vi "Tree Map to Tree Control Items.vi"(7 "Preserve Insertion Order? (F)":bool, 11 "Tree Map In":T2) -> (3 "Tree Control Items":T1(array[cluster]))   [LabVIEW 2020, in "Tree Map.lvlib"]
doc: "Translates the Tree Map representation into Tree Control Elements.\n\n<b>NOTE</b> - The order of elements is defined in alphabetical order, due to the implementation of Sets and Maps in LabVIEW. This effect only appears if there are 1M+ nodes with the same name under the same parent node. \nIf a different order of visualization is required, the user needs to access the array of Tree Control elements returned by this function and reorder the items using a custom algorithm.\n\n<b>Author:</b> Piotr Kruczkowski <PrimaryKey>\n<b>License:</b> NewBSD\n\nCopyright (c) 2019, National Instruments\nAll rights reserved.\n\nRedistribution and use in source and binary forms, with or without\nmodification, are permitted provided that the following conditions are met:\n1. Redistributions of source code must retain the above copyright\n notice, this list of conditions and the following disclaimer.\n2. Redistributions in binary form must reproduce the above copyright\n notice, this list of conditions and the following disclaimer in the\n documentation and/or other materials provided with the distribution.\n3. Neither the name of National Instruments nor the\n names of its contributors may be used to endorse or promote products\n derived from this software without specific prior written permission.\n\nTHIS SOFTWARE IS PROVIDED BY National Instruments ''AS IS'' AND ANY\nEXPRESS OR IMPLIED WARRANTIES, INCLUDING, BUT NOT LIMITED TO, THE IMPLIED\nWARRANTIES OF MERCHANTABILITY AND FITNESS FOR A PARTICULAR PURPOSE ARE\nDISCLAIMED. IN NO EVENT SHALL National Instruments BE LIABLE FOR ANY\nDIRECT, INDIRECT, INCIDENTAL, SPECIAL, EXEMPLARY, OR CONSEQUENTIAL DAMAGES\n(INCLUDING, BUT NOT LIMITED TO, PROCUREMENT OF SUBSTITUTE GOODS OR SERVICES;\nLOSS OF USE, DATA, OR PROFITS; OR BUSINESS INTERRUPTION) HOWEVER CAUSED AND\nON ANY THEORY OF LIABILITY, WHETHER IN CONTRACT, STRICT LIABILITY, OR TORT\n(INCLUDING NEGLIGENCE OR OTHERWISE) ARISING IN ANY WAY OUT OF THE USE OF THIS\nSOFTWARE, EVEN IF ADVISED OF THE POSSIBILITY OF SUCH DAMAGE."
uses:
  Tree Map.lvlib
  Tree Map Data.ctl
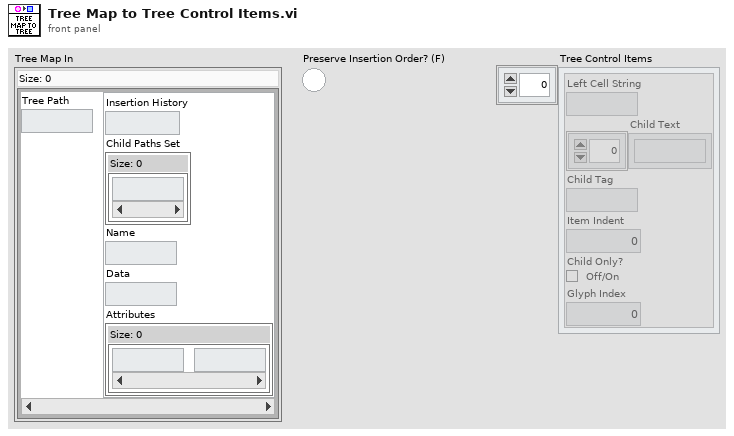
[diagram p1: front panel]
types:
  T1 = cluster{"Left Cell String":string, "Child Text":string[], "Child Tag":string, "Item Indent":i32, "Child Only?":bool, "Glyph Index":i32}[]
  T2 = typedef "Tree Map.lvlib/Tree Map Data.ctl" = map{string, cluster{"Insertion History":i32, "Child Paths Set":set{string}, "Name":string, "Data":string, "Attributes":map{string, string}}}
  T3 = cluster{"Insertion History":i32, "Left Cell String":string, "Child Text":string[], "Child Tag":string, "Item Indent":i32, "Child Only?":bool, "Glyph Index":i32}[]
  T4 = cluster{"Left Cell String":string, "Child Text":string[], "Child Tag":string, "Item Indent":i32, "Child Only?":bool, "Glyph Index":i32}
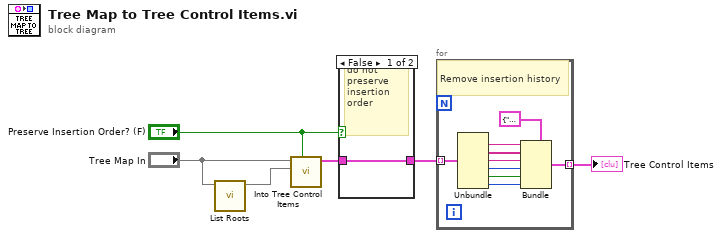
[diagram p0: block diagram]
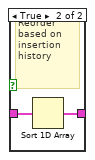
[diagram p2: hidden frame]
diagram:
  n1 = call "List Roots.vi"("Tree Map In"="Tree Map In") -> ("Unique Root Paths Set"=w5:set{string})  [unwired: 9 in, 1 out]
  n2 = call "Into Tree Control Items.vi"("Preserve Insertion Order? (F)"="Preserve Insertion Order? (F)", "Paths Set"=w5, "Tree Map In"="Tree Map In") -> ("Tree Control Item"=w4:T3)  [unwired: 8 in]
  n3 = case shown="False" "Preserve Insertion Order? (F)" {
    tunnel: w4 -> [w7 w9]
    tunnel: [w7 w8] -> w2
    frame False {
      # "do not preserve insertion order"
    }
    frame True {
      # "Reorder based on insertion history"
      n4 = Sort 1D Array(array=w9) -> (sorted array=w8:T3)
    }
  }
  n5 = for {
    tunnel: w2 -> [w18] mode=indexing
    tunnel: [w10] -> w3 mode=indexing
    # "Remove insertion history"
    n6 = Unbundle(w18) -> ("Left Cell String"=w16:string, "Child Text"=w15:string[], "Child Tag"=w14:string, "Item Indent"=w13:i32, "Child Only?"=w12:bool, "Glyph Index"=w11:i32)  [unwired: 1 out]
    n7 = Bundle(cluster=T4 {"Left Cell String"="", "Child Text"=[], "Child Tag"="", "Item Indent"=0, "Child Only?"=FALSE, "Glyph Index"=0} ("Tree Control Item"), "Left Cell String"=w16, "Child Text"=w15, "Child Tag"=w14, "Item Indent"=w13, "Child Only?"=w12, "Glyph Index"=w11) -> (w10:T4)
  }
  "Tree Control Items" <- w3
